vi "DAQmx Read (Counter U32 1Chan 1Samp).vi"(0 "task/channels in":refnum<k21>, 9 "timeout":dbl=10.0 format="%0.2f", 11 "error in":errorcluster) -> (4 "task out":refnum<k21>, 6 "data":u32, 15 "error out":errorcluster)   [LabVIEW 2020]
doc: "Reads a 32-bit unsigned integer sample from a counter task. Use an instance that reads 32-bit unsigned integers when NI-DAQmx returns counter samples unscaled, such as for event counting.\n\nIf the sample unit of your task cannot be represented by an integer, <B>data</B> is returned in the unit of clock ticks."
uses:
  nilvaiu.dll
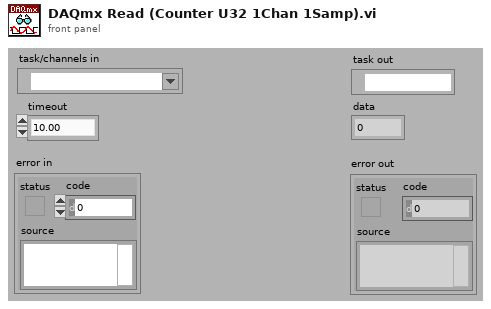
[diagram p1: front panel]
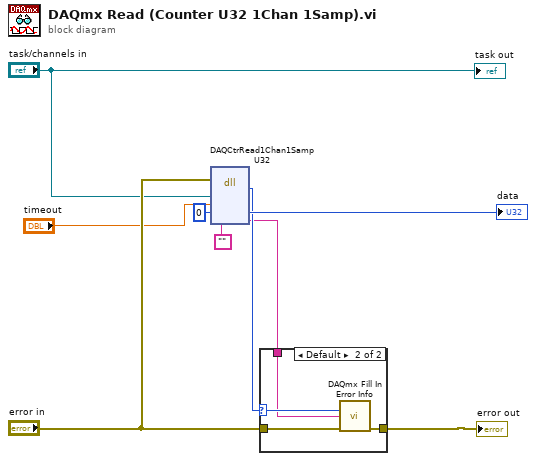
[diagram p0: block diagram]
diagram:
  n1 = dll-call lib="nilvaiu.*" fn="DAQCtrRead1Chan1SampU32"(error in="error in", "taskID"="task/channels in", "timeout"="timeout", "data"=u32 0, "extendedErrorInfo"="") -> (w4:i32, "data"=→"data":u32, "extendedErrorInfo"=w1:string)  [unwired: 3 in, 3 out]
  n2 = case shown="Default" w4 {
    selector: w4 -> [_ w12]
    tunnel: "error in" -> [w10 w14]
    tunnel: [w10 w13] -> w8
    tunnel: w1 -> [_ w11]
    frame 0 {
    }
    frame Default {
      n3 = call "DAQmx Fill In Error Info.vi"("status code"=w12, "extended error info"=w11, "error in"=w14) -> ("error out"=w13:errorcluster)  [unwired: 1 in, 11 out]
    }
  }
  "error out" <- w8
  "task out" <- "task/channels in"
